vi "niSE Disconnect.vi"(8 "error in (no error)":errorcluster, 10 "disconnect_specification":string, 11 "Session Factory in":refnum<class "Session Factory.lvclass">) -> (0 "error out":errorcluster, 3 "Session Factory out":refnum<class "Session Factory.lvclass">)   [LabVIEW 2021, in "NI Session Management niSE.lvlib" / "Session Factory.lvclass"]
uses:
  Session Factory.lvclass
  basic_switch_executive_driver_client/RPC Messages/nise_DisconnectInfo.ctl
  basic_switch_executive_driver_client/RPC Messages/nise_SessionInformation.ctl
  <vilib>/Plug-In SDKs/Clients/Session Management V1/Session Reservation/Initialize and Close Session Behavior.ctl
  Session Factory.lvclass/Session Factory.ctl
  basic_switch_executive_driver_client/basic_switch_executive_driver_client.lvlib
  <vilib>/Plug-In SDKs/Clients/Session Management V1/Session Reservation/Session Reservation.lvclass
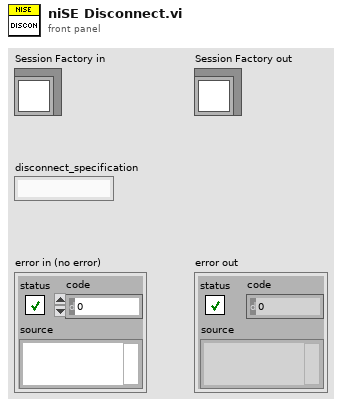
[diagram p1: front panel]
types:
  T1 = typedef "basic_switch_executive_driver_client.lvlib/nise_DisconnectInfo.ctl" = cluster{"disconnect_specification":string, "session_info":T2}
  T2 = typedef "basic_switch_executive_driver_client.lvlib/nise_SessionInformation.ctl" = cluster{"session_id":u32, "initialize_and_close_session_behavior":T3}
  T3 = typedef "NI Session Management V1 Client.lvlib/Session Reservation.lvclass/Initialize and Close Session Behavior.ctl" = enum16{"Auto", "Initialize and Close", "Attach and Detach", "Initialize and Detach", "Attach and Close"}
  T4 = typedef "grpc-lvsupport-release.lvlib/grpcId.ctl" = u64
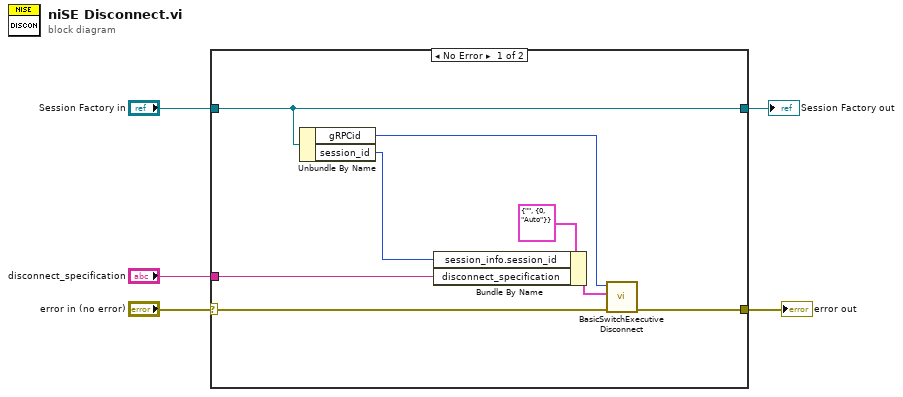
[diagram p0: block diagram]
diagram:
  n1 = case shown="No Error" "error in (no error)" {
    selector: "error in (no error)" -> [w13 w15]
    tunnel: [w12 w15] -> w4
    tunnel: [w11 w14] -> w2
    tunnel: "Session Factory in" -> [w11 w14]
    tunnel: "disconnect_specification" -> [w7 _]
    frame No Error {
      n2 = Unbundle By Name(w11) -> ("gRPCid"=w10:T4, "session_id"=w6:u32)
      n3 = Bundle By Name(cluster=T1 {"disconnect_specification"="", "session_info"={"session_id"=0, "initialize_and_close_session_behavior"=enum."Auto"}} ("Request Data"), "session_info.session_id"=w6, "disconnect_specification"=w7) -> (w8:T1)
      n4 = call "BasicSwitchExecutive Disconnect.vi"("error in"=w13, "Request Data"=w8, "gRPC ID"=w10) -> ("error out"=w12:errorcluster)  [unwired: 6 in, 2 out]
    }
    frame Error {
    }
  }
  "error out" <- w4
  "Session Factory out" <- w2
